vi "Send Notification.vi"(8 "error in (no error)":errorcluster, 9 "Notification Data":variant, 10 "Notification Action":T1, 11 "navX - Interface in":refnum<class "navX - Interface.lvclass">) -> (0 "error out":errorcluster, 3 "navX - Interface out":refnum<class "navX - Interface.lvclass">)   [LabVIEW 2015, in "navX Library v3.lvlib" / "navX - Interface.lvclass"]
uses:
  navX - Interface.lvclass
  _TypeDefs/NotificationActionsTypeDef.ctl
  _TypeDefs/NotificationPacketTypeDef.ctl
  navX - Interface.lvclass/navX - Interface.ctl
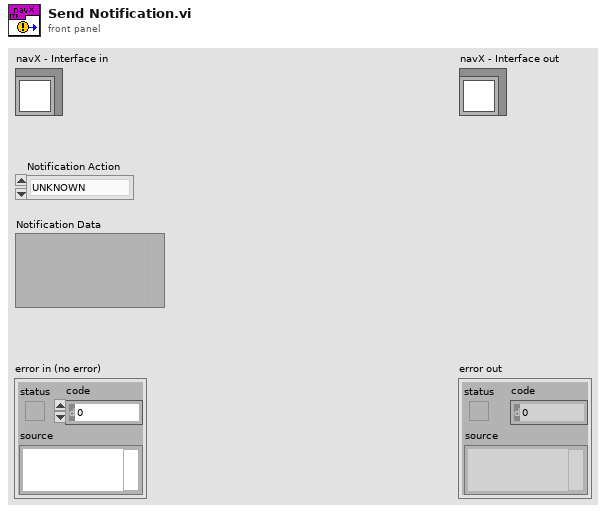
[diagram p1: front panel]
types:
  T1 = typedef "navX Library v3.lvlib/navX - Interface.lvclass/NotificationActionsTypeDef.ctl" = enum16{"UNKNOWN", "Stop Processing Loop", "Reconfigure", "Zero"}
  T2 = typedef "navX Library v3.lvlib/navX - Interface.lvclass/NotificationPacketTypeDef.ctl" = cluster{"Notification Action":T1, "Notification Data":variant}
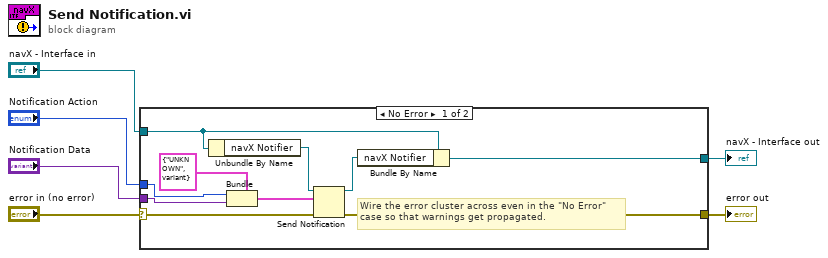
[diagram p0: block diagram]
diagram:
  n1 = case shown="No Error" "error in (no error)" {
    selector: "error in (no error)" -> [w8 w18]
    tunnel: [w7 w18] -> w5
    tunnel: [w16 w17] -> w3
    tunnel: "navX - Interface in" -> [w15 w17]
    tunnel: "Notification Action" -> [w11 _]
    tunnel: "Notification Data" -> [w10 _]
    frame No Error {
      # "Wire the error cluster across even in the \"No Error\"\ncase so that warnings get propagated."
      n2 = Unbundle By Name(w15) -> ("navX Notifier"=w14:refnum<notifier>)
      n3 = Bundle(cluster=T2 {"Notification Action"=enum."UNKNOWN", "Notification Data"=variant} ("Notification Packet"), "Notification Action"=w11, "Notification Data"=w10) -> (w9:T2)
      n4 = Send Notification(notification=w9, notifier=w14, error in (no error)=w8) -> (notifier out=w13:refnum<notifier>, error out=w7:errorcluster)
      n5 = Bundle By Name(cluster=w15, "navX Notifier"=w13) -> (w16:refnum<class "navX - Interface.lvclass">)
    }
    frame Error {
    }
  }
  "error out" <- w5
  "navX - Interface out" <- w3
